vi "DP - Read desired position.vi"(2 "error in":errorcluster, 3 "Axis":i8=1 min=1 max=6 step=1, 4 "Address / Port":i16=1 min=1 max=31 step=1) -> (0 "error out":errorcluster, 1 "Read desired position":dbl format="%.5f")   [LabVIEW 2014]
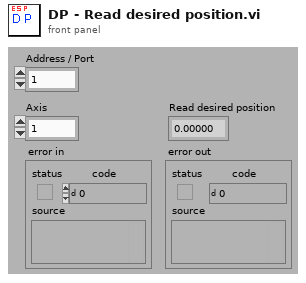
[diagram p1: front panel]
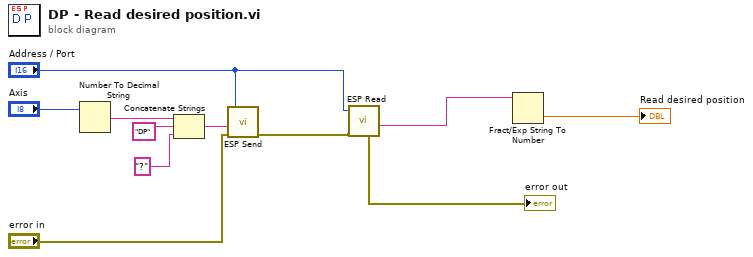
[diagram p0: block diagram]
diagram:
  n1 = Number To Decimal String(number="Axis") -> (decimal integer string=w10:string)  [unwired: 1 in]
  n2 = Concatenate Strings(w10, "DP" ("Substring"), "?" ("Substring")) -> (w8:string)
  n3 = call "ESP Send.vi"("Address / Port"="Address / Port", "Command String"=w8, "error in"="error in") -> ("error out"=w3:errorcluster)  [unwired: 5 in]
  n4 = call "ESP Read.vi"("Address / Port"="Address / Port", "error in"=w3) -> ("error out"=→"error out":errorcluster, "Response String"=w5:string)  [unwired: 5 in]
  n5 = Fract/Exp String To Number(string=w5) -> (number=→"Read desired position":dbl)  [unwired: 3 in, 1 out]
